vi "get channel value by id.vi"(8 "error in (no error)":errorcluster, 10 "id":string, 11 "configuration file cluster in":T1) -> (0 "error out":errorcluster, 1 "found?":bool, 2 "channel":T9, 3 "configuration file cluster out":T1)   [LabVIEW 2017, in "DSF Configuration API v1.0.0.lvlib"]
uses:
  DSF Configuration API v1.0.0.lvlib
  get item index by id/get channel index by id.vi
  Controls/dsf configuration file/1.0.0/DSF Channel.ctl
  File API/DSFConfig.lvlib
  Controls/dsf configuration file/1.0.0/DSF Transfer.ctl
  Controls/dsf configuration file/1.0.0/dsf timing.ctl
  Controls/dsf configuration file/1.0.0/DSF Group.ctl
  Controls/dsf configuration file/1.0.0/DSF Plugin.ctl
  Controls/dsf configuration file/1.0.0/Version Info.ctl
  Controls/dsf configuration file/1.0.0/DSF Settings.ctl
  Controls/dsf configuration file/1.0.0/DSF Config.ctl
  Controls/dsf configuration file/1.0.0/DSF Channel Info.ctl
  Controls/dsf configuration file/1.0.0/DSF Settings Info.ctl
  Controls/dsf configuration file/1.0.0/DSF Transfer Info.ctl
  File API/DSF Plugin Info.ctl
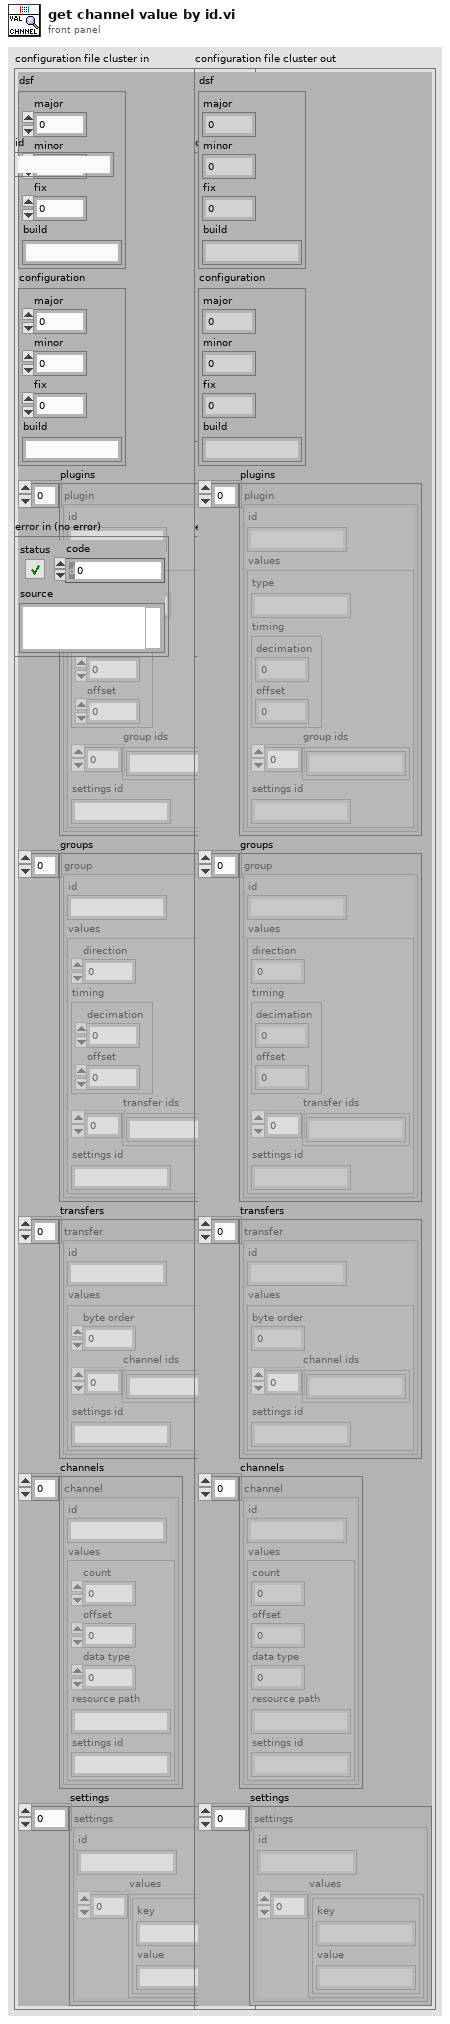
[diagram p1: front panel]
types:
  T1 = typedef "DSFConfig.lvlib/DSF Config.ctl" = cluster{"dsf":T2, "configuration":T2, "plugins":T3[], "groups":T6[], "transfers":T7[], "channels":T9[], "settings":T11[]}
  T2 = typedef "DSFConfig.lvlib/Version Info.ctl" = cluster{"major":u32, "minor":u32, "fix":u32, "build":string}
  T3 = typedef "DSFConfig.lvlib/DSF Plugin.ctl" = cluster{"id":string, "values":T4}
  T4 = typedef "DSFConfig.lvlib/DSF Plugin Info.ctl" = cluster{"type":string, "timing":T5, "group ids":string[], "settings id":string}
  T5 = typedef "DSFConfig.lvlib/dsf timing.ctl" = cluster{"decimation":i32, "offset":i32}
  T6 = typedef "DSFConfig.lvlib/DSF Group.ctl" = cluster{"id":string, "values":cluster{"direction":i32, "timing":T5, "transfer ids":string[], "settings id":string}}
  T7 = typedef "DSFConfig.lvlib/DSF Transfer.ctl" = cluster{"id":string, "values":T8}
  T8 = typedef "DSFConfig.lvlib/DSF Transfer Info.ctl" = cluster{"byte order":i32, "channel ids":string[], "settings id":string}
  T9 = typedef "DSFConfig.lvlib/DSF Channel.ctl" = cluster{"id":string, "values":T10}
  T10 = typedef "DSFConfig.lvlib/DSF Channel Info.ctl" = cluster{"count":i32, "offset":i32, "data type":i32, "resource path":string, "settings id":string}
  T11 = typedef "DSFConfig.lvlib/DSF Settings.ctl" = cluster{"id":string, "values":T12}
  T12 = typedef "DSFConfig.lvlib/DSF Settings Info.ctl" = cluster{"key":string, "value":string}[]
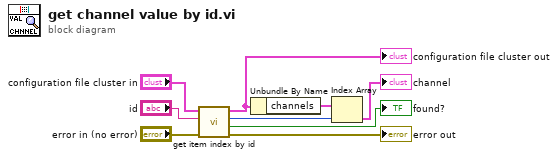
[diagram p0: block diagram]
diagram:
  n1 = call-poly "get item index by id.vi"("error in (no error)"="error in (no error)", "id"="id", "configuration file cluster in"="configuration file cluster in") -> ("error out"=→"error out":errorcluster, "found?"=→"found?":bool, "index"=w4:i32, "configuration file cluster out"=w8:T1)  [unwired: 5 in]
  "configuration file cluster out" <- w8
  n2 = Unbundle By Name(w8) -> ("channels"=w5:T9[])
  n3 = Index Array(array=w5, index=w4) -> (element=→"channel":T9)
